vi "Dialog_Enter Loop Iterations.vi"(8 "Error In":errorcluster) -> (0 "Error Out":errorcluster, 2 "Cancelled?":bool, 3 "Macro Command":string)   [LabVIEW 2012]
doc: "SciScan 1.2 160622\nThis VI has no controls.\nThis is a dummy whihc runs when user selects a macro command which does not require any arguments"
uses:
  Custom Controls and Typedefs/Macro_CommandStruct.ctl
  Custom Controls and Typedefs/Macro_Action_List.ctl
  Custom Controls and Typedefs/Macro_ArgumentStruct.ctl
panel:
  out "Macro Commands":T1
  in  "Cancel Button":bool
  in  "OK Button":bool
  in  "Iter.No":dbl=1.0 min=1.0 step=1.0
  # "Enter the number of iterations for the LOOP"
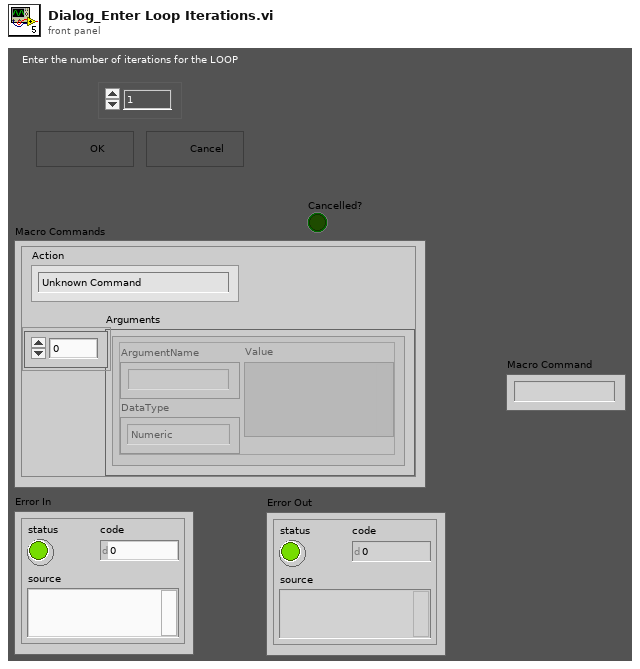
[diagram p1: front panel]
types:
  T1 = typedef "Macro_CommandStruct.ctl" = cluster{"Action":T2, "Arguments":T3[]}
  T2 = typedef "Macro_Action_List.ctl" = enum16{"Unknown Command", "2D.Frame.Scan", "2D.Line.Scan", "Load.Settings.File", "Move.To.Position", "Pause", "Z.Stack", "LOOP.Start", "LOOP.End", "Record", "Fast.Z", "Generic", "Slow.Z", "Tiling", "Preset.End"}
  T3 = typedef "Macro_ArgumentStruct.ctl" = cluster{"ArgumentName":string, "DataType":enum16{"Numeric", "String"}, "Value":variant}
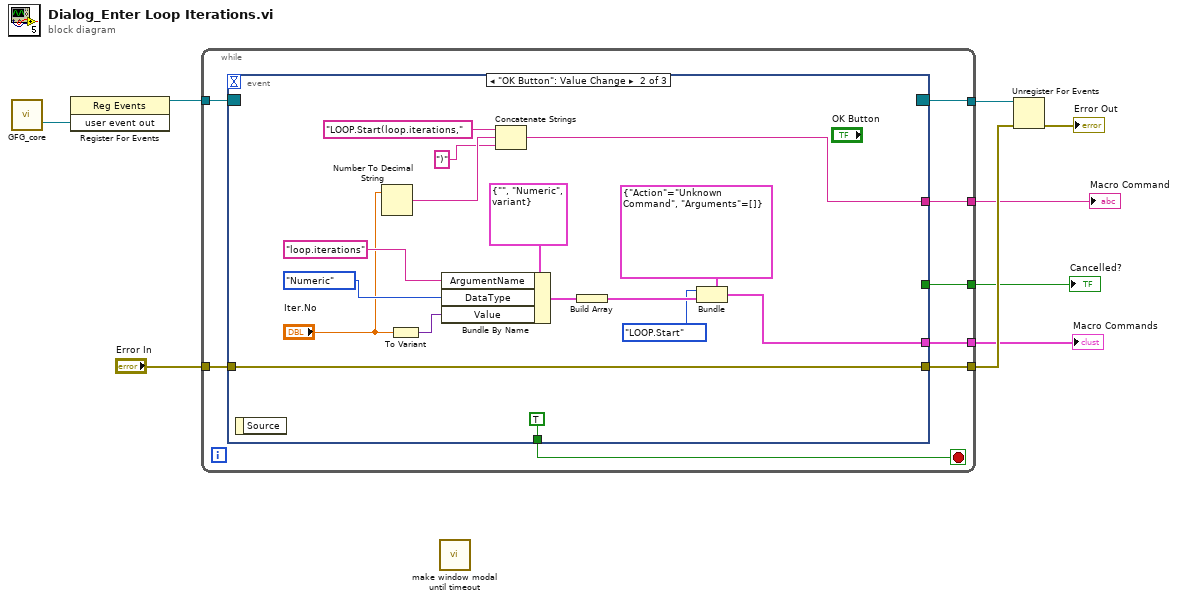
[diagram p0: block diagram]
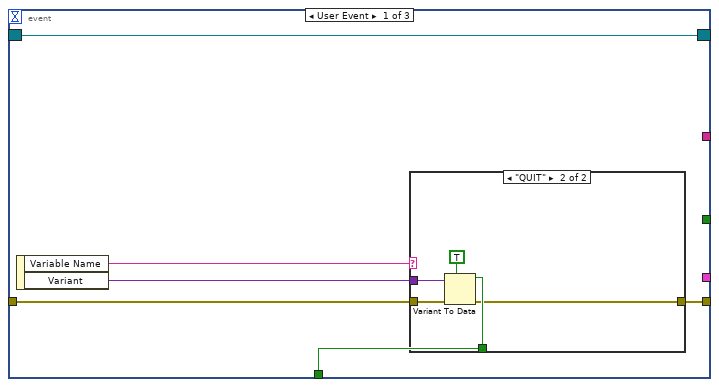
[diagram p2: hidden frame]
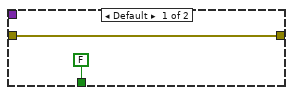
[diagram p3: hidden frame]
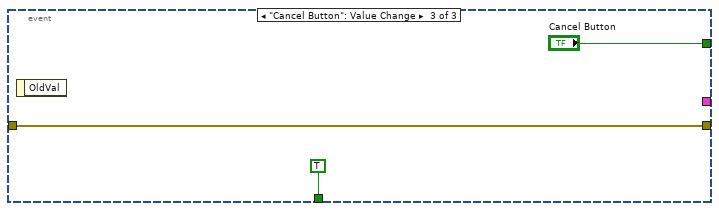
[diagram p4: hidden frame]
diagram:
  n1 = call "GFG_core.vi"() -> ("user event out"=w9:refnum<user-event>)  [unwired: 13 in, 6 out]
  n2 = register-events(w9) -> (reference out=w8:refnum<event-registration>)  [unwired: 2 in, 1 out]
  n3 = while {
    tunnel: w8 -> [w17]
    tunnel: [w16] -> w7
    tunnel: "Error In" -> [w14]
    tunnel: [w13] -> w5
    tunnel: [w12] -> w3
    tunnel: [w11] -> w2
    tunnel: [w10] -> w1
    stop <- w15 stop-if-true
    n4 = event shown="[1] \"OK Button\": Value Change" {
      selector: w17 -> [w23 _ _]
      dyn-events: [w23 _ _] -> w16
      timeout: _ -> [_ _ _]
      tunnel: [w20 TRUE TRUE] -> w15
      tunnel: w14 -> [w19 w37 w48]
      tunnel: [w18 w37 w48] -> w13
      tunnel: [_ w38 _] -> w12
      tunnel: [_ _ "Cancel Button"] -> w11
      tunnel: [_ w31 _] -> w10
      event User Event {
        n5 = event-data() -> ("Variable Name"=w22:string, "Variant"=w21:variant)  [unwired: 1 in]
        n6 = case shown="\"QUIT\"" w22 {
          tunnel: w21 -> [_ w29]
          tunnel: [FALSE w28] -> w20
          tunnel: w19 -> [w24 w27]
          tunnel: [w24 w26] -> w18
          frame Default {
          }
          frame "QUIT" {
            n7 = Variant To Data(error in=w27, type=TRUE, Variant=w29) -> (data=w28:bool, error out=w26:errorcluster)
          }
        }
      }
      event "OK Button": Value Change {
        n8 = event-data() -> ()  [unwired: 1 in, 1 out]
        n9 = Number To Decimal String(number="Iter.No") -> (decimal integer string=w33:string)  [unwired: 1 in]
        n10 = To Variant(anything="Iter.No") -> (Variant=w44:variant)
        n11 = Bundle By Name(cluster=T3 {"ArgumentName"="", "DataType"=enum."Numeric", "Value"=variant} ("Arguments"), "ArgumentName"="loop.iterations", "DataType"=enum16{"Numeric", "String"}."Numeric", "Value"=w44) -> (w41:T3)
        n12 = Concatenate Strings("LOOP.Start(loop.iterations," ("ArgumentName"), w33, ")" ("ArgumentName")) -> (w31:string)
        n13 = Build Array(w41) -> (w40:T3[])
        n14 = Bundle(cluster=T1 {"Action"=enum."Unknown Command", "Arguments"=[]} ("Macro Commands"), "Action"=Macro_Action_List."LOOP.Start", "Arguments"=w40) -> (w38:T1)
      }
      event "Cancel Button": Value Change {
        n15 = event-data() -> ()  [unwired: 1 in, 1 out]
      }
    }
  }
  "Macro Commands" <- w3
  "Cancelled?" <- w2
  "Macro Command" <- w1
  n16 = call "make window modal until timeout.vi"() -> ()  [unwired: 12 in]
  n17 = Unregister For Events(event registration refnum=w7, error in=w5) -> (error out=→"Error Out":errorcluster)
